vi "Power Function Simulator.vi"(9 "Function Parameters":cluster{"Prefactor":dbl, "Power":dbl}={"Prefactor"=5.0, "Power"=4.0}, 10 "Digitizing Parameters":T2={"Number of Samples"=100, "Lower Limit"=0.0, "Upper Limit"=10.0}) -> (2 "Output Cluster":T1)   [LabVIEW 2017]
uses:
  <vilib>/imath/engines/lvmath2/RunTimeEngine/Managers/WorkSpace/UID Generator.vi
  <vilib>/imath/engines/lvmath2/RunTimeEngine/RunTimeType/NIMS_RunTimeType_From StrictType (excl LVString).vi
  <instcachedir>/0/NIMS_RunTimeType_From StrictType (excl LVString)_1019F277F0A747EDBCA0F6C52CA54500.lvgen/NIMS_RunTimeType_From StrictType (excl LVString)_1019F277F0A747EDBCA0F6C52CA54500_000.vi
  <vilib>/imath/engines/lvmath2/RunTimeEngine/LocalVariableDefStatement/MC_LocalVariableDefStatement_Display.vi
  <vilib>/imath/engines/lvmath2/RunTimeEngine/RangeToken/NIMS_Range.vi
  <instcachedir>/0/NIMS_Range_69CB9AAD882742A19CF7E739BE79952C.lvgen/NIMS_Range_69CB9AAD882742A19CF7E739BE79952C_000.vi
  <vilib>/imathl/engines/lvmath/Functions/Error Handling/Create Error.vi
  <vilib>/imath/engines/lvmath2/RunTimeEngine/ArithmeticOperatorToken/NIMS_ArithmeticOperator_power(S).vi
  <instcachedir>/0/NIMS_ArithmeticOperator_power(S)_86B1D76B77564424912EAFCCCC7488ED.lvgen/NIMS_ArithmeticOperator_power(S)_86B1D76B77564424912EAFCCCC7488ED_014.vi
  <vilib>/imath/engines/lvmath2/RunTimeEngine/Managers/SymbolTable/Clear UID.vi
  <vilib>/imath/engines/lvmath2/RunTimeEngine/NodeEndStatement/NIMS_NodeEndStatement_Output.vi
  <instcachedir>/0/NIMS_NodeEndStatement_Output_53EC0D466D134D7ABD903AC30B43404B.lvgen/NIMS_NodeEndStatement_Output_53EC0D466D134D7ABD903AC30B43404B_001.vi
  <instcachedir>/0/NIMS_NodeEndStatement_Output_53EC0D466D134D7ABD903AC30B43404B.lvgen/NIMS_NodeEndStatement_Output_53EC0D466D134D7ABD903AC30B43404B_000.vi
  <instcachedir>/0/NIMS_NodeEndStatement_Output_53EC0D466D134D7ABD903AC30B43404B.lvgen/NIMS_NodeEndStatement_Output_53EC0D466D134D7ABD903AC30B43404B_005.vi
  <vilib>/imath/engines/lvmath2/RunTimeEngine/ErrorHandling/NIMS_Finalize Error.vi
  <vilib>/imath/engines/lvmath2/RunTimeEngine/Managers/SymbolTable/NIMS_WorkSpace.lvlib
panel:
  out "XY Graph":cluster{"x":dbl[], "y":dbl[]}(graph)
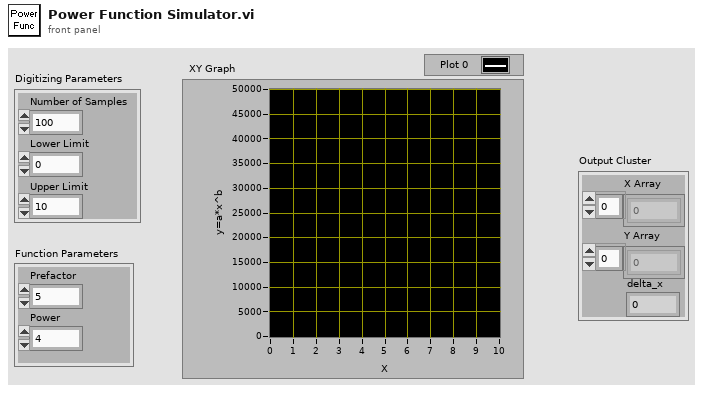
[diagram p1: front panel]
types:
  T1 = cluster{"X Array":dbl[], "Y Array":dbl[], "delta_x":dbl}
  T2 = cluster{"Number of Samples":i32, "Lower Limit":dbl, "Upper Limit":dbl}
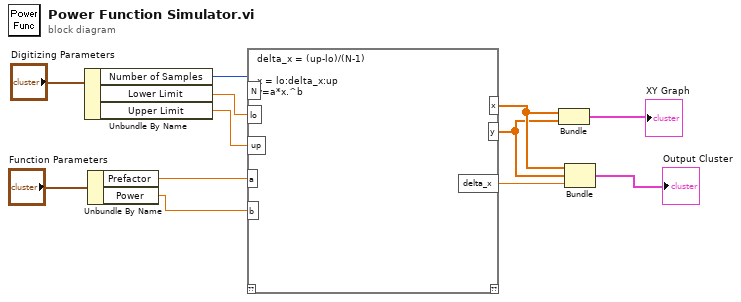
[diagram p0: block diagram]
diagram:
  n1 = Unbundle By Name("Digitizing Parameters") -> ("Number of Samples"=w10:i32, "Lower Limit"=w9:dbl, "Upper Limit"=w8:dbl)
  n2 = Unbundle By Name("Function Parameters") -> ("Prefactor"=w7:dbl, "Power"=w6:dbl)
  n3 = mathscript code="delta_x = (up-lo)/(N-1)\n\nx = lo:delta_x:up\ny=a*x.^b"("N"=w10, "lo"=w9, "up"=w8, "a"=w7, "b"=w6) -> ("x"=w4:dbl[], "y"=w3:cdb[], "delta_x"=w2:dbl)  [unwired: 1 in, 1 out]
  n4 = Bundle("x"=w4, "y"=w3) -> (→"XY Graph":cluster{"x":dbl[], "y":cdb[]})  [unwired: 1 in]
  n5 = Bundle("x"=w4, "y"=w3, "delta_x"=w2) -> (→"Output Cluster":cluster{"x":dbl[], "y":cdb[], "delta_x":dbl})  [unwired: 1 in]
